vi "Sno4BarArm.vi"(1 "Pot Set Point":dbl=0.4, 2 "Desired Height Above Ground":dbl=0.4, 3 "PID gains":T13={"proportional gain (Kc)"=25.0, "integral time (Ti, min)"=0.0, "derivative time (Td, min)"=0.0}, 4 "PotDevRef":T10, 5 "MotorControlDevRef":T1={"DeviceStatus"={"status"=FALSE, "code"=0, "source"=""}, "Type"=enum."PWM", "PWM"={"Controller"=enum."Controller 1", "PWM Channel"=enum."Invalid", "DeadBand"={"Name"="", "maxPositivePwm"=0, "minPositivePwm"=0, "centerPwm"=0, "maxNegativePwm"=0, "minNegativePwm"=0, "angularRange"=0}}, "CAN"={"Device Number"=0, "Control Mode"=enum."Percent VBus", "Semaphore"=refnum, "Max Vout"=12.0, "TalonSRX Control Mode"=enum."Percent VBus"}, "Invert"=FALSE, "TransformRef"=refnum, "InvTransformRef"=refnum}) -> (0 "error out":errorcluster)   [LabVIEW 2014]
uses:
  <vilib>/Rock Robotics/WPI/Potentiometer/WPI_PotentiometerDevRef.ctl
  <vilib>/Rock Robotics/SystemInterfaces/Typedef/FPGA_TypedefAnalogModule.ctl
  <vilib>/Rock Robotics/SystemInterfaces/AI/FPGA_AIChannel.ctl
  <vilib>/Rock Robotics/WPI/MotorControl/WPI_MotorControlDeviceRef.ctl
  <vilib>/Rock Robotics/WPI/MotorControl/WPI_MotorControlType.ctl
  <vilib>/Rock Robotics/SystemInterfaces/Typedef/FPGA_TypedefDigitalModule.ctl
  <vilib>/Rock Robotics/SystemInterfaces/DIO/FPGA_DIOPWMChannel.ctl
  <vilib>/Rock Robotics/WPI/PWM/WPI_PWMDeadband.ctl
  <vilib>/Rock Robotics/WPI/CAN/Jaguar/SubVIs/WPI_CANJaguar_ControlMode.ctl
  <vilib>/Rock Robotics/WPI/CAN/TalonSRX/WPI_CANTalonSRX_APIControlMode.ctl
  <vilib>/Rock Robotics/WPI/PWM/WPI_PWMTransform_ConPane.ctl
  <vilib>/addons/control/pid/pid.llb/PID Control Input Filter (DBL).vi
  <vilib>/addons/control/pid/pid.llb/PID (DBL).vi
  <vilib>/addons/control/pid/NI_PID_pid.lvlib
  <vilib>/Analysis/NI_AALPro.lvlib
panel:
  out "Waveform Chart":dbl(graph)
  out "Error Small?":bool
  out "Pot Error":dbl
  out "Current Pot Value":dbl
  out "Set Point":dbl
  out "Current Time":u32
  out "Start Time":u32
  out "New Pot Setpoint":dbl=0.2 format="%0.2f"
  in  "Meters Above the Ground":dbl[](array[numeric])=[0.0, 0.4, 0.8, 1.2, 1.6, 2.0] format="%0.2f"
  in  "Pot Values":dbl[](array[numeric])=[0.0, 0.2, 0.4, 0.5, 0.55, 0.6, 0.65, 0.7, 0.75, 0.8, 0.9] format="%0.2f"
  out "Filter Output":dbl format="%.2f"
  out "motor output":dbl
  in  "output range":cluster{"output high":dbl, "output low":dbl}={"output high"=1.0, "output low"=-1.0}
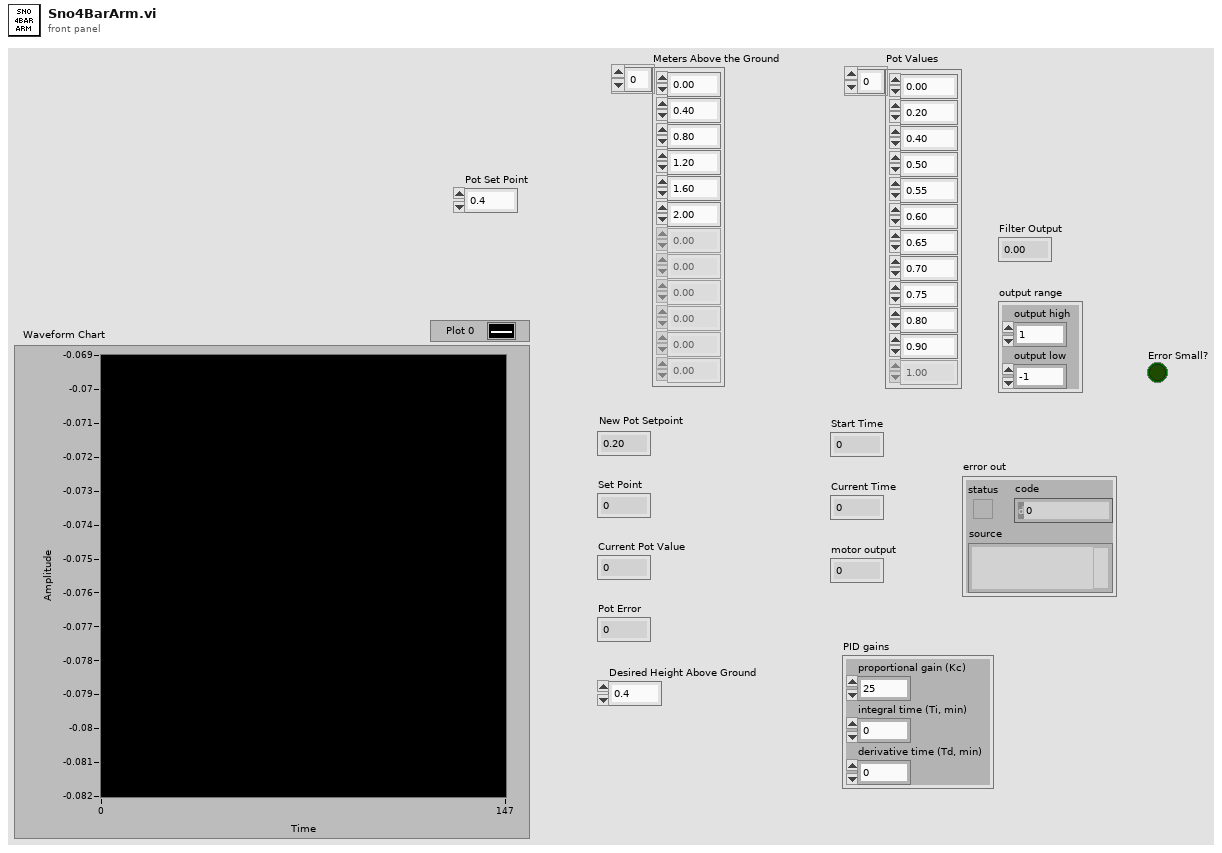
[diagram p1: front panel]
types:
  T1 = typedef "WPI_MotorControlDeviceRef.ctl" = cluster{"DeviceStatus":errorcluster, "Type":T2, "PWM":cluster{"Controller":T3, "PWM Channel":T4, "DeadBand":T5}, "CAN":cluster{"Device Number":u8, "Control Mode":T6, "Semaphore":T7, "Max Vout":dbl, "TalonSRX Control Mode":T8}, "Invert":bool, "TransformRef":T9, "InvTransformRef":T9}
  T2 = typedef "WPI_MotorControlType.ctl" = enum16{"PWM", "CAN", "CANTalonSRX"}
  T3 = typedef "FPGA_TypedefDigitalModule.ctl" = enum16{"Controller 1"}
  T4 = typedef "FPGA_DIOPWMChannel.ctl" = enum8{"PWM 0", "PWM 1", "PWM 2", "PWM 3", "PWM 4", "PWM 5", "PWM 6", "PWM 7", "PWM 8", "PWM 9", "PWM MXP 0", "PWM MXP 1", "PWM MXP 2", "PWM MXP 3", "PWM MXP 4", "PWM MXP 5", "PWM MXP 6", "PWM MXP 7", "PWM MXP 8", "PWM MXP 9", "Invalid"}
  T5 = typedef "WPI_PWMDeadband.ctl" = cluster{"Name":string, "maxPositivePwm":i32, "minPositivePwm":i32, "centerPwm":i32, "maxNegativePwm":i32, "minNegativePwm":i32, "angularRange":u16}
  T6 = typedef "WPI_CANJaguar_ControlMode.ctl" = enum8{"Percent VBus", "Current", "Speed", "Position", "Voltage"}
  T7 = typedef "Semaphore RefNum" = refnum<k1>
  T8 = typedef "WPI_CANTalonSRX_APIControlMode.ctl" = enum8{"Percent VBus", "Speed", "Position", "Slave", "Unchanged / Invalid"}
  T9 = typedef "WPI_PWMTransform_ConPane.ctl" = refnum<vi>
  T10 = typedef "WPI_PotentiometerDevRef.ctl" = cluster{"DevStatus":errorcluster, "Controller":T11, "Analog Channel":T12, "Invert Output":bool}
  T11 = typedef "FPGA_TypedefAnalogModule.ctl" = enum16{"Controller 1"}
  T12 = typedef "FPGA_AIChannel.ctl" = enum8{"AI 0", "AI 1", "AI 2", "AI 3", "AI MXP 0", "AI MXP 1", "AI MXP 2", "AI MXP 3", "Invalid"}
  T13 = cluster{"proportional gain (Kc)":dbl, "integral time (Ti, min)":dbl, "derivative time (Td, min)":dbl}
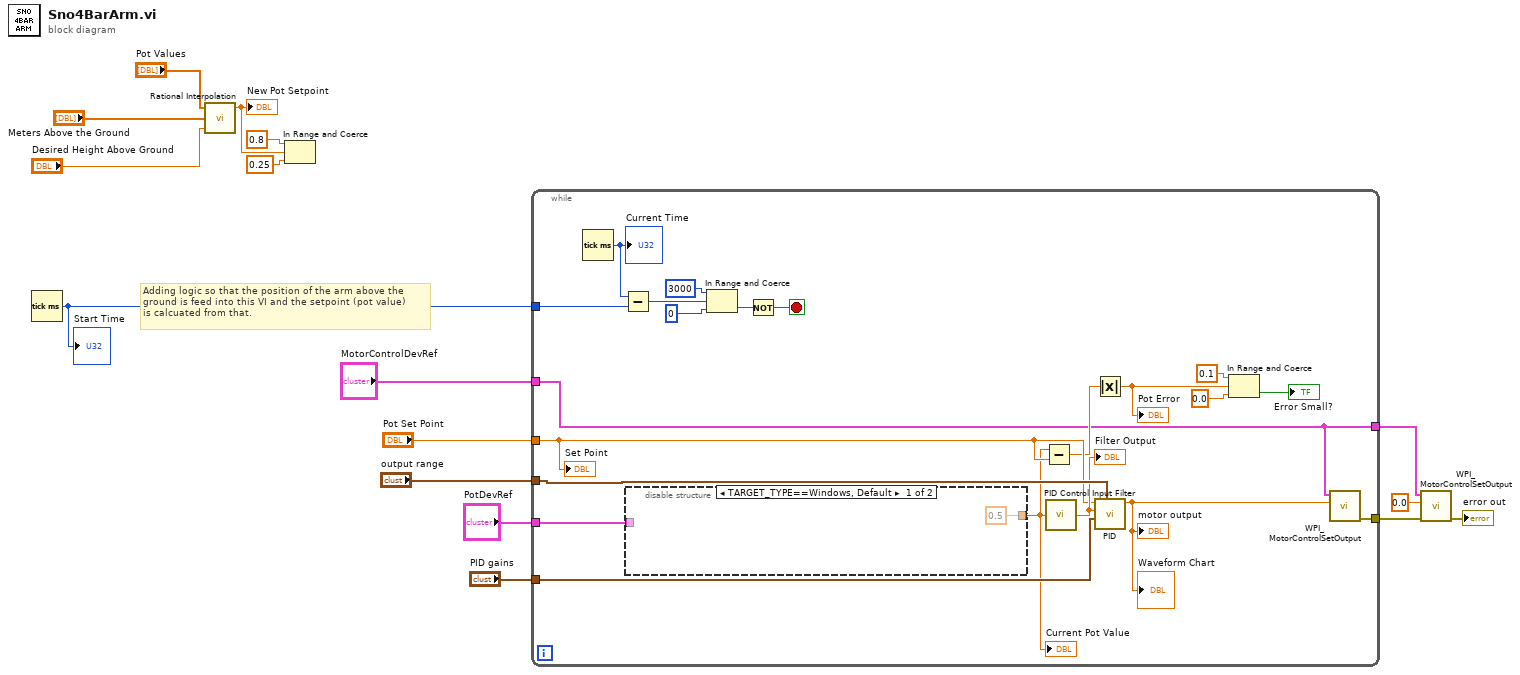
[diagram p0: block diagram]
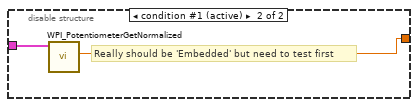
[diagram p2: hidden frame]
diagram:
  # "Adding logic so that the position of the arm above the\nground is feed into this VI and the setpoint (pot value)\nis calcuated from that."
  n1 = Tick Count (ms)() -> (millisecond timer value=w11:u32)
  "Start Time" <- w11
  n2 = call <vilib>:"Rational Interpolation.vi"("x value"="Desired Height Above Ground", "X"="Meters Above the Ground", "Y"="Pot Values") -> ("interpolation value"=w4:dbl)  [unwired: 2 out]
  "New Pot Setpoint" <- w4
  n3 = In Range and Coerce(upper limit=0.8, x=w4, lower limit=0.25) -> ()  [unwired: 2 out]
  n4 = while {
    tunnel: "PotDevRef" -> [w20]
    tunnel: "MotorControlDevRef" -> [w17]
    tunnel: "Pot Set Point" -> [w27]
    tunnel: "output range" -> [w37]
    tunnel: "PID gains" -> [w36]
    tunnel: w11 -> [w33]
    tunnel: [w18] -> w10
    tunnel: [w17] -> w8
    stop <- w28 stop-if-true
    n5 = Tick Count (ms)() -> (millisecond timer value=w34:u32)
    "Current Time" <- w34
    n6 = Subtract(x=w34, y=w33) -> (x-y=w30:u32)
    n7 = disable-structure shown="TARGET_TYPE==Windows, Default" {
      disable-tunnel: w20 -> [_ w40]
      disable-tunnel: [0.5 w39] -> w19
      frame condition #0 {
      }
      frame condition #1 (active) {
        # "Really should be 'Embedded' but need to test first"
        n8 = call <vilib>:"WPI_PotentiometerGetNormalized.vi"("PotDevRef"=w40) -> ("Normalized Value"=w39:dbl)  [unwired: 8 in, 2 out]
      }
    }
    "Current Pot Value" <- w19
    n9 = In Range and Coerce(upper limit=u32 3000, x=w30, lower limit=u32 0) -> (In Range?=w29:bool)  [unwired: 1 out]
    n10 = Not(x=w29) -> (.not. x?=w28:bool)
    n11 = Subtract(x=w19, y=w27) -> (x-y=w26:dbl)
    n12 = call-poly <vilib>:"PID Control Input Filter.vi"("input"=w19) -> ("output"=w35:dbl)  [unwired: 4 in]
    "Filter Output" <- w35
    n13 = Absolute Value(x=w26) -> (abs(x)=w23:dbl)
    "Pot Error" <- w23
    n14 = call-poly <vilib>:"PID.vi"("output range"=w37, "PID gains"=w36, "process variable"=w35, "setpoint"=w27) -> ("output"=w21:dbl)  [unwired: 6 in, 1 out]
    "motor output" <- w21
    "Waveform Chart" <- w21
    n15 = In Range and Coerce(upper limit=0.1, x=w23, lower limit=0.0) -> (In Range?=→"Error Small?":bool)  [unwired: 1 out]
    n16 = call <vilib>:"WPI_MotorControlSetOutput.vi"("Output"=w21, "MotorControlDevRef"=w17) -> ("error out"=w18:errorcluster)  [unwired: 7 in, 2 out]
    "Set Point" <- w27
  }
  n17 = call <vilib>:"WPI_MotorControlSetOutput.vi"("error in (no error)"=w10, "Output"=0.0, "MotorControlDevRef"=w8) -> ("error out"=→"error out":errorcluster)  [unwired: 6 in, 2 out]
